vi "Generate 3D Picture.vi"(7 "Tip Model File (.wrl)":path=path "E:/labview_proj/AFM tip/AFMtip LAO-STO-Si.wrl", 8 "error in (no error)":errorcluster, 9 "Show Axis":bool, 10 "X Length":sgl=4.0, 11 "Y Length":sgl=4.0) -> (0 "error out":errorcluster, 1 "Canvas":refnum<vi>, 2 "Tip":refnum<vi>, 3 "SceneObject out":refnum<vi>)   [LabVIEW 2020]
doc: "This VI creates the 3D picture by creating an axis and adding the tip and the canvas."
uses:
  <vilib>/picture/3D Picture Control/Object/Create Object (name).vi
  <vilib>/picture/3D Picture Control/Object/Add Object (reference).vi
  <vilib>/picture/3D Picture Control/NI_3D Picture Control.lvlib
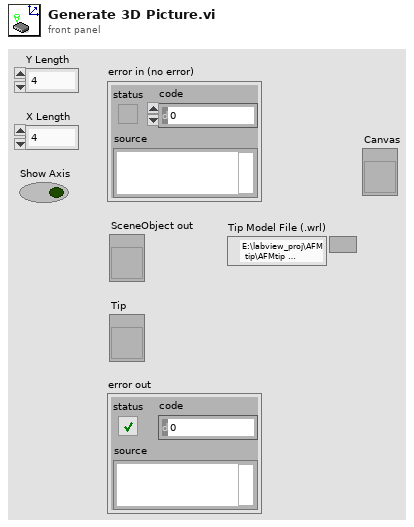
[diagram p1: front panel]
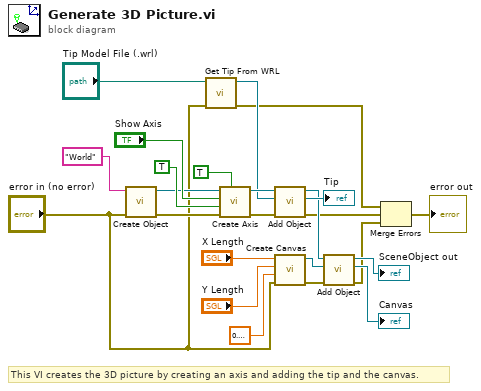
[diagram p0: block diagram]
diagram:
  # "This VI creates the 3D picture by creating an axis and adding the tip and the canvas."
  n1 = call-poly <vilib>:"Create Object.vi"("error in (no error)"="error in (no error)", "Name"="World") -> ("error out"=w15:errorcluster, "Scene:New Object"=w16:refnum<vi>)  [unwired: 8 in]
  n2 = call "Get Tip From WRL.vi"("error in (no error)"="error in (no error)", "Tip Model File (.wrl)"="Tip Model File (.wrl)") -> ("error out"=w6:errorcluster, "SceneObject out"=w13:refnum<vi>)  [unwired: 8 in]
  n3 = call "Create Axis.vi"("Axis label?"=TRUE, "error in (no error)"=w15, "Half plane?"=TRUE, "Show Axis"="Show Axis", "SceneObject in"=w16) -> ("error out"=w8:errorcluster, "SceneObject out"=w14:refnum<vi>)  [unwired: 5 in]
  n4 = call-poly <vilib>:"Add Object.vi"("error in (no error)"=w8, "New Object In"=w13, "Scene Object In"=w14) -> ("error out"=w5:errorcluster, "New Object Out"=→"Tip":refnum<vi>, "Scene Object Out"=w10:refnum<vi>)  [unwired: 6 in]
  n5 = call "Create Canvas.vi"("error in (no error)"="error in (no error)", "Z"=sgl 0.1 ("Length Z"), "Y"="Y Length", "X"="X Length") -> ("error out"=w2:errorcluster, "SceneObject out"=w1:refnum<vi>)  [unwired: 6 in]
  n6 = call-poly <vilib>:"Add Object.vi"("error in (no error)"=w2, "New Object In"=w1, "Scene Object In"=w10) -> ("error out"=w4:errorcluster, "New Object Out"=→"Canvas":refnum<vi>, "Scene Object Out"=→"SceneObject out":refnum<vi>)  [unwired: 6 in]
  n7 = Merge Errors(w6, w5, w4) -> (→"error out":errorcluster)
